vi "Sub_online_LEMP_Update_LAB-formula.vi"(1 "Effected DOF":i32, 2 "Mode count":i32, 3 "LEMP":T1) -> (0 "Updated Eigenvalues":dbl[](array[numeric]))   [LabVIEW 2021]
panel:
  # "Inputs"
  # "Output"
  # "This Vi the minimal possible operations to prep data for the secular equation solver, then sails to \"C\" to use the secular equation solver dll and returns the updated Eigenvalues. While offline, the prior Eigenvalues, the squares of each value in the prior Eigenvectors the equivalent stiffness change for the rolle are each attained. The modes used and the Effected DOF are constants provided at runtime. The index and  truncation operations are miniscules time uses however \"technically\" if memory and speed are absolutely critical then truncation of the eigenvalues and eigenvectors could be performed at initialization losing the modecount \"dynamic\" variation at runtime functionality. The memory time and memory saved is O(n+n*(n-m)) where n is the number of nodes and m is the number of modes.\n\n              - Alexander Vereen AFRL Summer scholars 2022"
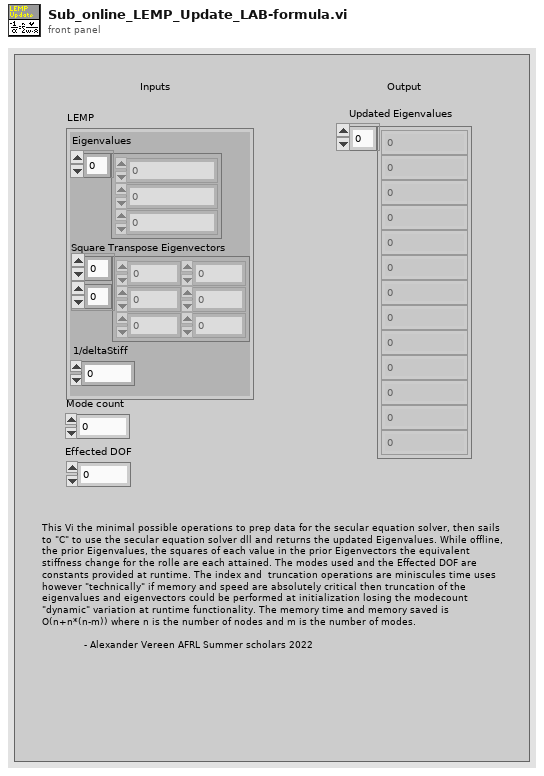
[diagram p1: front panel]
types:
  T1 = cluster{"Eigenvalues":dbl[], "Square Transpose Eigenvectors":dbl[][], "1/deltaStiff":dbl}
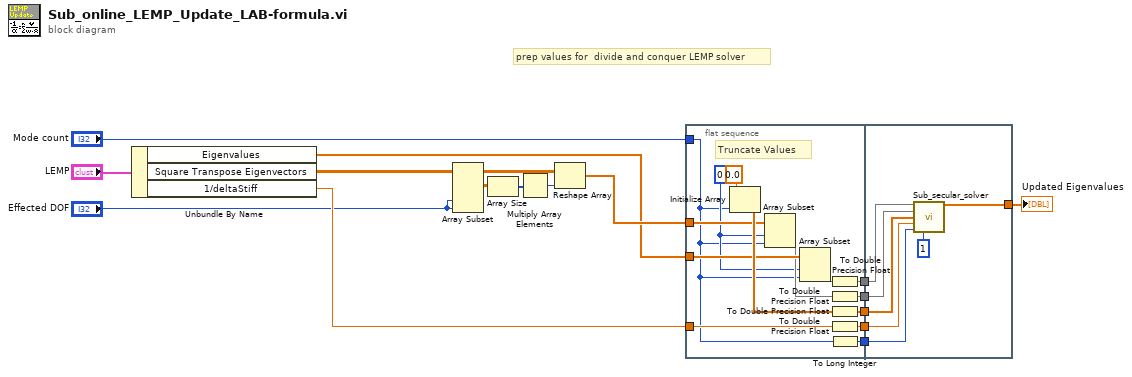
[diagram p0: block diagram]
diagram:
  # "prep values for  divide and conquer LEMP solver"
  n1 = Unbundle By Name("LEMP") -> ("Eigenvalues"=w3:dbl[], "Square Transpose Eigenvectors"=w4:dbl[][], "1/deltaStiff"=w2:dbl)
  n2 = Array Subset(array=w4, index (col)="Effected DOF", length (col)="Effected DOF") -> (w8:dbl[][])  [unwired: 2 in]
  n3 = Array Size(array=w8) -> (size(s)=w11:i32[])
  n4 = Multiply Array Elements(1:w11) -> (0:w10:i32)
  n5 = Reshape Array(w8, w10) -> (w9:dbl[])
  n6 = flat-sequence {
    tunnel: w9 -> [w27]
    tunnel: w3 -> [w26]
    tunnel: w2 -> [w30]
    tunnel: "Mode count" -> [w21]
    tunnel: [w22] -> w16
    tunnel: [w20] -> w15
    tunnel: [w18] -> w13
    tunnel: [w19] -> w12
    tunnel: [w17] -> w14
    tunnel: w16 -> [w33]
    tunnel: w15 -> [w32]
    tunnel: w14 -> [w37]
    tunnel: w13 -> [w36]
    tunnel: w12 -> [w35]
    tunnel: [w34] -> w7
    frame #0 {
      w24 = 0
      # "Truncate Values"
      n7 = Initialize Array(0.0, w21) -> (w28:dbl[])
      n8 = Array Subset(array=w27, index=w24, length=w21) -> (w25:dbl[])
      n9 = Array Subset(array=w26, index=w24, length=w21) -> (w23:dbl[])
      n10 = To Double Precision Float(number=w23) -> (double precision float=w22:dbl[])
      n11 = To Double Precision Float(number=w25) -> (double precision float=w20:dbl[])
      n12 = To Double Precision Float(number=w28) -> (double precision float=w19:dbl[])
      n13 = To Double Precision Float(number=w30) -> (double precision float=w18:dbl)
      n14 = To Long Integer(number=w21) -> (32bit integer=w17:i32)
    }
    frame #1 {
      n15 = call "Sub_secular_solver.vi"("Eigenvalues"=w33, "Transpose Eigenvectors"=w32, "Empty Solution Array"=w35, "Inverse Delta in Stiffness"=w36, "Total Modes"=w37, "Total Corrections"=1) -> ("New Eigenvalues"=w34:dbl[])  [unwired: 9 in]
    }
  }
  "Updated Eigenvalues" <- w7
